vi "Write Parameters.vi"(4 "error in (no error)":errorcluster, 6 "rangeParams":T1, 7 "appended path":path) -> (0 "error out":errorcluster)   [LabVIEW 2015]
uses:
  <vilib>/Utility/config.llb/Write Key (Double).vi
  <vilib>/Utility/config.llb/NI_LVConfig.lvlib
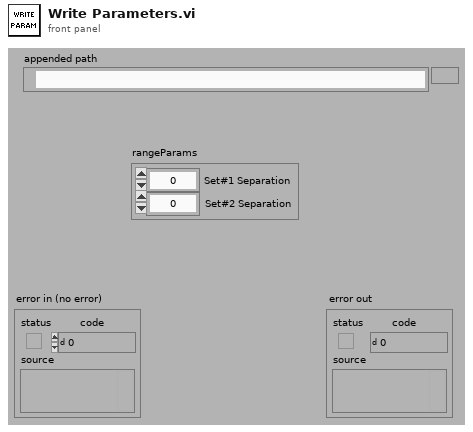
[diagram p1: front panel]
types:
  T1 = cluster{"Set#1 Separation":sgl, "Set#2 Separation ":sgl}
  T2 = typedef "NI_LVConfig.lvlib/Config Data RefNum.ctl" = refnum<k1>
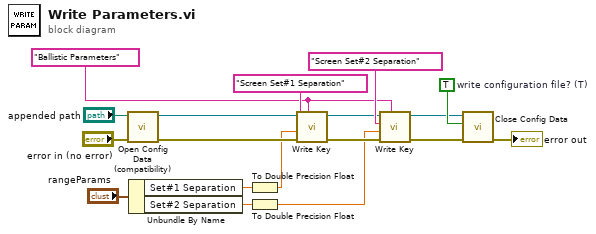
[diagram p0: block diagram]
diagram:
  w18 = TRUE  # write configuration file? (T)
  w10 = "Ballistic Parameters"
  n1 = call <vilib>:"Open Config Data (compatibility).vi"("error in (no error)"="error in (no error)", "configuration file path"="appended path") -> ("error out"=w9:errorcluster, "refnum"=w8:T2)  [unwired: 7 in, 1 out]
  n2 = Unbundle By Name("rangeParams") -> ("Set#1 Separation"=w4:sgl, "Set#2 Separation"=w3:sgl)
  n3 = To Double Precision Float(number=w4) -> (double precision float=w2:dbl)
  n4 = To Double Precision Float(number=w3) -> (double precision float=w1:dbl)
  n5 = call-poly <vilib>:"Write Key.vi"("section"=w10, "error in (no error)"=w9, "value"=w2, "key"="Screen Set#1 Separation", "refnum"=w8) -> ("error out"=w11:errorcluster, "refnum out"=w12:T2)  [unwired: 4 in, 1 out]
  n6 = call-poly <vilib>:"Write Key.vi"("section"=w10, "error in (no error)"=w11, "value"=w1, "key"="Screen Set#2 Separation", "refnum"=w12) -> ("error out"=w7:errorcluster, "refnum out"=w6:T2)  [unwired: 4 in, 1 out]
  n7 = call <vilib>:"Close Config Data.vi"("error in (no error)"=w7, "write file if changed (T)"=w18, "refnum"=w6) -> ("error out"=→"error out":errorcluster)  [unwired: 8 out]
